vi "color scale.vi"(11 "Array":u32[](array[colorbox])=[16711680, 16772608, 6618880, 3381759, 16860, 10420479, 16448250]) -> (3 "appended array 2":dbl[][](array[numeric]))   [LabVIEW 2016]
uses:
  <userlib>/LevyLab/Graph Utilities/graph_utilities.lvclass
panel:
  in  "Array 3":u32[](array[colorbox])=[16711680, 16772608, 6618880, 3381759, 16860, 10420479, 11479807, 12539135, 13598463, 14657791, 15717631, 16448250]
  in  "Array 2":u32[](array[colorbox])=[16711680, 16772608, 6618880, 3381759, 16860, 10420479, 12539135, 14657791, 16448250]
  in  "file (use dialog)":path=path "C:/Users/ansom/Desktop"
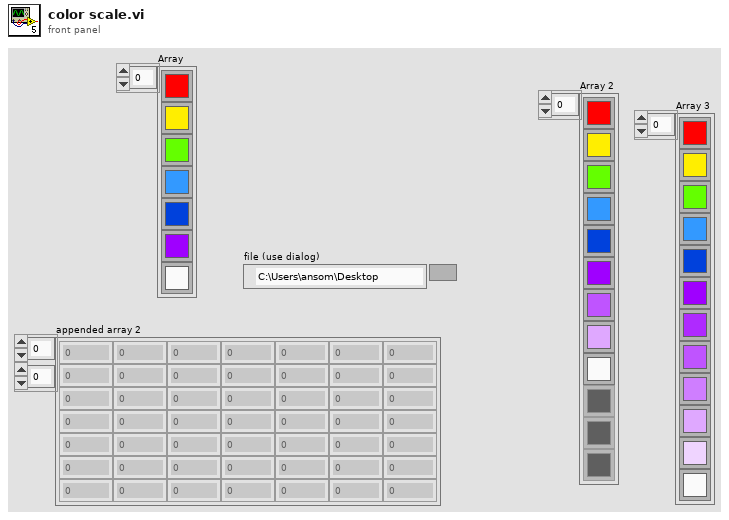
[diagram p1: front panel]
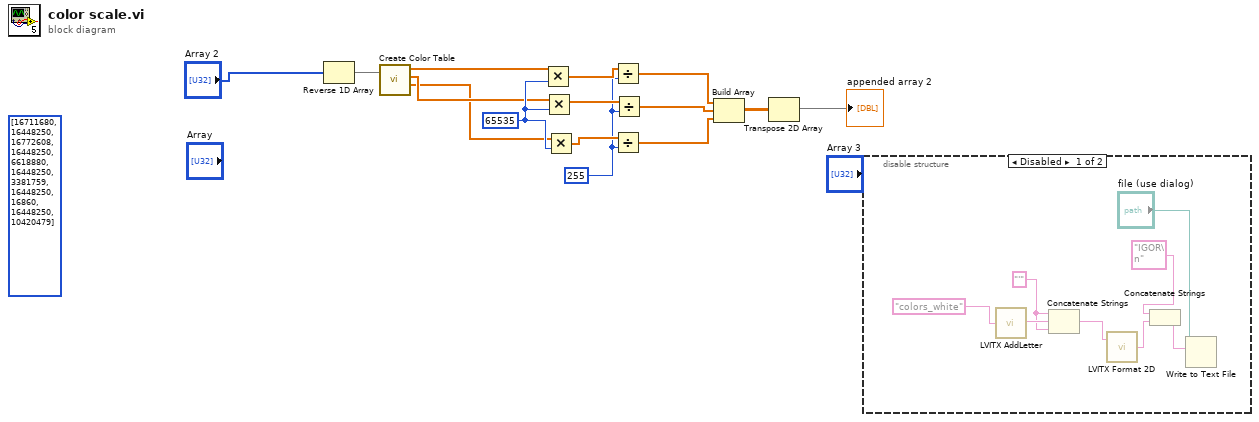
[diagram p0: block diagram]
diagram:
  w11 = 255
  w15 = 65535
  (unwired) u32[] [16711680, 16448250, 16772608, 16448250, 6618880, 16448250, 3381759, 16448250, 16860, 16448250, 10420479] ("Array")
  n1 = Reverse 1D Array(array="Array 2") -> (reversed array=w3:u32[])
  n2 = call <userlib>:"Create Color Table.vi"("Colors []"=w3) -> ("R []"=w10:dbl[], "G []"=w9:dbl[], "B []"=w8:dbl[])  [unwired: 1 in, 1 out]
  n3 = Multiply(x=w10, y=w15) -> (x*y=w14:dbl[])
  n4 = Multiply(x=w9, y=w15) -> (x*y=w13:dbl[])
  n5 = Multiply(x=w8, y=w15) -> (x*y=w12:dbl[])
  n6 = Divide(x=w14, y=w11) -> (x/y=w7:dbl[])
  n7 = Divide(x=w12, y=w11) -> (x/y=w5:dbl[])
  n8 = Divide(x=w13, y=w11) -> (x/y=w6:dbl[])
  n9 = Build Array(w7, w6, w5) -> (w4:dbl[][])
  n10 = Transpose 2D Array(2D array=w4) -> (transposed array=→"appended array 2":dbl[][])
  n11 = disable-structure shown="Disabled" {
    frame Disabled {
      w20 = "'" ("string")
      n12 = call <userlib>:"LVITX AddLetter.vi"("String"="colors_white" ("2D Array name")) -> ("output string"=w21:string)
      n13 = Concatenate Strings(w20, w21, w20) -> (w19:string)
      n14 = call <userlib>:"LVITX Format 2D.vi"("2D Array name"=w19) -> ("String"=w17:string)  [unwired: 1 in]
      n15 = Concatenate Strings("IGOR\n", w17) -> (w16:string)
      n16 = Write to Text File(file (use dialog)="file (use dialog)", text=w16) -> ()  [unwired: 1 in, 4 out]
    }
    frame Enabled {
    }
  }
